vi "timer check for animation.vi"(10 "timer (ms)":dbl, 11 "refresh time (ms)":dbl) -> (3 "Enum":T1)   [LabVIEW 2020]
uses:
  controls/animation logic enum 1.ctl
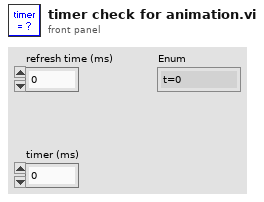
[diagram p1: front panel]
types:
  T1 = typedef "animation logic enum 1.ctl" = enum16{"t=0", "t>=max", "0<t<max"}
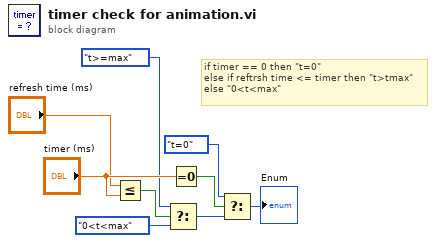
[diagram p0: block diagram]
diagram:
  # "if timer == 0 then \"t=0\"\nelse if reftrsh time <= timer then \"t>tmax\"\nelse \"0<t<max\""
  n1 = Less Or Equal?(x="refresh time (ms)", y="timer (ms)") -> (x <= y?=w4:bool)
  n2 = Select(t=animation_logic_enum_1."t>=max", s=w4, f=animation_logic_enum_1."0<t<max") -> (s? t:f=w6:T1)
  n3 = Equal To 0?(x="timer (ms)") -> (x = 0?=w2:bool)
  n4 = Select(t=animation_logic_enum_1."t=0", s=w2, f=w6) -> (s? t:f=→"Enum":T1)
